vi "readBin(U8).vi"(9 "Size":i32=1, 10 "Offset":i32=48, 11 "Buffer IN":string) -> (1 "int":u8, 2 "Offset+size":i32, 3 "Buffer OUT":string)   [LabVIEW 2017, in "HEKAdat.lvclass"]
uses:
  HEKAdat.lvclass
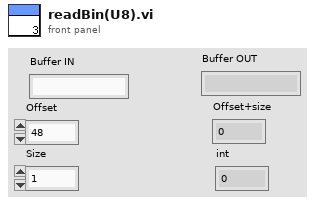
[diagram p1: front panel]
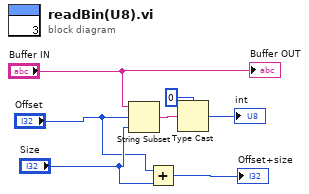
[diagram p0: block diagram]
diagram:
  n1 = String Subset(string="Buffer IN", offset (0)="Offset", length (rest)="Size") -> (substring=w5:string)
  n2 = Add(x="Offset", y="Size") -> (x+y=→"Offset+size":i32)
  n3 = Type Cast(type=u8 0 ("오프셋(0)"), x=w5) -> (*(type *) &x=→"int":u8)
  "Buffer OUT" <- "Buffer IN"
